vi "GEOM_GetWCSDirectives.vi"(10 "hdrs":T1[](array[typedef])=[{"name"="TRIMSEC", "directives"={"coords"="amp", "reference"="phys", "xarea"="xdatastart:xdataend", "yarea"="ydatastart:ydataend", "order"="fits"}, "comment"="Good section", "amptype"=enum."ALL", "ampid"=FALSE, "detid"=FALSE, "unbin"=FALSE}, {"name"="DETSEC", "directives"={"coords"="fpa", "reference"="pix", "xarea"="xdatastart:xdataend", "yarea"="ydatastart:ydataend", "order"="fits"}, "comment"="Detector display tile", "amptype"=enum."ALL", "ampid"=FALSE, "detid"=FALSE, "unbin"=FALSE}, {"name"="CCDSEC", "directives"={"coords"="det", "reference"="pix", "xarea"="xdatastart:xdataend", "yarea"="ydatastart:ydataend", "order"="fits"}, "comment"="CCD section to display", "amptype"=enum."ALL", "ampid"=FALSE, "detid"=FALSE, "unbin"=FALSE}, {"name"="AMPSEC", "directives"={"coords"="amp", "reference"="pix", "xarea"="xdatastart:xdataend", "yarea"="ydatastart:ydataend", "order"="readout"}, "comment"="CCD section in read order", "amptype"=enum."ALL", "ampid"=FALSE, "detid"=FALSE, "unbin"=FALSE}, {"name"="DATASEC", "directives"={"coords"="amp", "reference"="phys", "xarea"="xdatastart:xdataend", "yarea"="ydatastart:ydataend", "order"="fits"}, "comment"="Data section to display", "amptype"=enum."ALL", "ampid"=FALSE, "detid"=FALSE, "unbin"=FALSE}, {"name"="BIASSEC", "directives"={"coords"="amp", "reference"="phys", "xarea"="xposstart:xposend", "yarea"="ydatastart:ydataend", "order"="fits"}, "comment"="Overscan", "amptype"=enum."ALL", "ampid"=FALSE, "detid"=FALSE, "unbin"=FALSE}, {"name"="PRESEC", "directives"={"coords"="amp", "reference"="phys", "xarea"="xprestart:xpreend", "yarea"="ydatastart:ydataend", "order"="fits"}, "comment"="Prescan", "amptype"=enum."ALL", "ampid"=FALSE, "detid"=FALSE, "unbin"=FALSE}, {"name"="POSTSEC", "directives"={"coords"="amp", "reference"="phys", "xarea"="xdatastart:xdataend", "yarea"="yposstart:yposend", "order"="fits"}, "comment"="Postscan", "amptype"=enum."ALL", "ampid"=FALSE, "detid"=FALSE, "unbin"=FALSE}]) -> (2 "directives out":string)   [LabVIEW 2016]
uses:
  Headers/GEOM_HdrSec.ctl
  Headers/GEOM_CoorSys.ctl
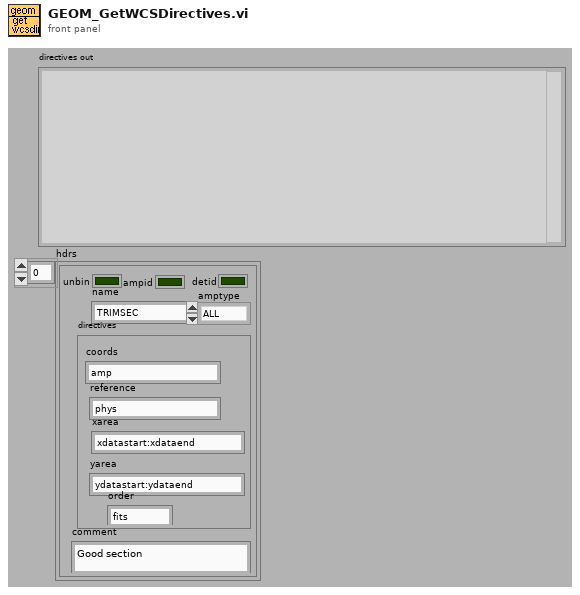
[diagram p1: front panel]
types:
  T1 = typedef "GEOM_HdrSec.ctl" = cluster{"name":string, "directives":T2, "comment":string, "amptype":enum16{"LL", "LR", "UL", "UR", "ALL", "LEFT", "RIGHT", "UPPER", "LOWER"}, "ampid":bool, "detid":bool, "unbin":bool}
  T2 = typedef "GEOM_CoorSys.ctl" = cluster{"coords":string, "reference":string, "xarea":string, "yarea":string, "order":string}
  T3 = enum16{"LL", "LR", "UL", "UR", "ALL", "LEFT", "RIGHT", "UPPER", "LOWER"}
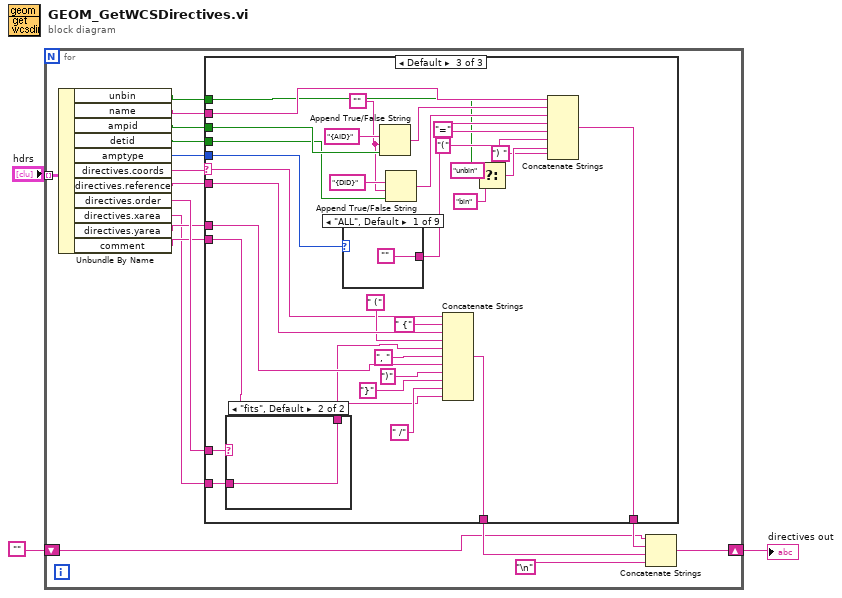
[diagram p0: block diagram]
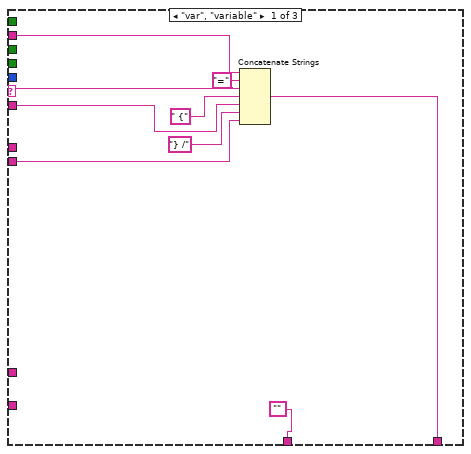
[diagram p2: hidden frame]
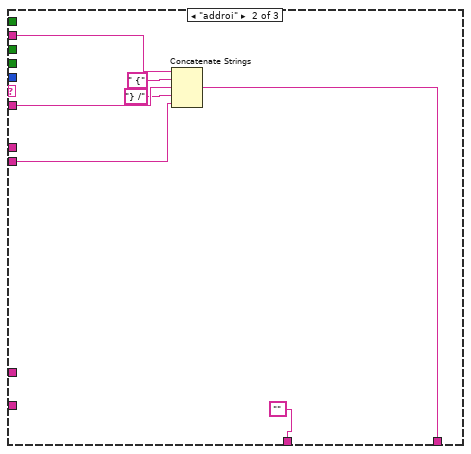
[diagram p3: hidden frame]
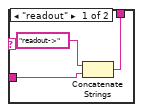
[diagram p4: hidden frame]
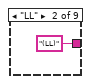
[diagram p5: hidden frame]
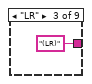
[diagram p6: hidden frame]
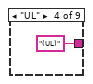
[diagram p7: hidden frame]
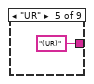
[diagram p8: hidden frame]
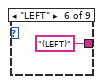
[diagram p9: hidden frame]
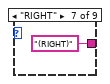
[diagram p10: hidden frame]
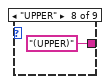
[diagram p11: hidden frame]
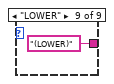
[diagram p12: hidden frame]
diagram:
  n1 = for {
    shift-right: [w11] -> w2
    shift-left: "" -> [w6]
    tunnel: "hdrs" -> [w8] mode=indexing
    n2 = Unbundle By Name(w8) -> ("unbin"=w7:bool, "name"=w18:string, "ampid"=w20:bool, "detid"=w19:bool, "amptype"=w17:T3, "directives.coords"=w4:string, "directives.reference"=w16:string, "directives.order"=w15:string, "directives.xarea"=w5:string, "directives.yarea"=w10:string, "comment"=w9:string)
    n3 = case shown="Default" w4 {
      selector: w4 -> [w25 _ w37]
      tunnel: w20 -> [_ _ w68]
      tunnel: w19 -> [_ _ w65]
      tunnel: w18 -> [w27 w35 w63]
      tunnel: w17 -> [_ _ w60]
      tunnel: w16 -> [w23 w33 w56]
      tunnel: w15 -> [_ _ w55]
      tunnel: [w28 w30 w54] -> w14
      tunnel: ["" "" w53] -> w13
      tunnel: w10 -> [_ _ w50]
      tunnel: w9 -> [w21 w31 w46]
      tunnel: w7 -> [_ _ w44]
      tunnel: w5 -> [_ _ w39]
      frame "var", "variable" {
        n4 = Concatenate Strings(w27, "=" ("string"), w25, " {" ("string"), w23, "} /" ("string"), w21) -> (w28:string)
      }
      frame "addroi" {
        n5 = Concatenate Strings(w35, " {" ("string"), w33, "} /" ("string"), w31) -> (w30:string)
      }
      frame Default {
        w64 = ""
        n6 = case shown="\"fits\", Default" w55 {
          tunnel: w39 -> [w70 w72]
          tunnel: [w69 w72] -> w38
          frame "readout" {
            n7 = Concatenate Strings("readout->", w70) -> (w69:string)
          }
          frame "fits", Default {
          }
        }
        n8 = case shown="\"ALL\", Default" w60 {
          tunnel: ["" "(LL)" "(LR)" "(UL)" "(UR)" "(LEFT)" "(RIGHT)" "(UPPER)" "(LOWER)"] -> w59
          frame "ALL", Default {
          }
          frame "LL" {
          }
          frame "LR" {
          }
          frame "UL" {
          }
          frame "UR" {
          }
          frame "LEFT" {
          }
          frame "RIGHT" {
          }
          frame "UPPER" {
          }
          frame "LOWER" {
          }
        }
        n9 = Append True/False String(1:w68, 2:w64, 3:"{AID}" ("true string")) -> (0:w62:string)  [unwired: 1 out]
        n10 = Append True/False String(1:w65, 2:w64, 3:"{DID}" ("true string")) -> (0:w61:string)  [unwired: 1 out]
        n11 = Concatenate Strings(w37, " {" ("string"), w56, " (" ("string"), w38, ", " ("string"), w50, ")" ("string"), "}" ("string"), " /" ("string"), w46) -> (w53:string)
        n12 = Select(t="unbin", s=w44, f="bin") -> (s? t:f=w41:string)
        n13 = Concatenate Strings(w63, w62, w61, w59, "=" ("string"), "(" ("string"), w41, ") " ("string")) -> (w54:string)
      }
    }
    n14 = Concatenate Strings(w6, w14, w13, "\n") -> (w11:string)
  }
  "directives out" <- w2
